vi "Is SPI Channel Ready for Next Transaction.vi"(8 "error in":errorcluster, 11 "Private Data In":T1={"DLU To SPI Engine Data FIFO"="DLU To SPI Engine Data", "SPI Engine to DLU Data FIFO"="SPI Engine to DLU Data", "Data to SPI Engine (Cache) Register"="Data to SPI Engine (Cache)", "SPI PHY Settings to SPI Engine (Cahche) Register"="SPI PHY Settings to SPI Engine (Cache)"}) -> (0 "error out":errorcluster, 1 "SPI Channel Ready":bool, 3 "Private Data Out":T1={"DLU To SPI Engine Data FIFO"="DLU To SPI Engine Data", "SPI Engine to DLU Data FIFO"="SPI Engine to DLU Data", "Data to SPI Engine (Cache) Register"="Data to SPI Engine (Cache)", "SPI PHY Settings to SPI Engine (Cahche) Register"="SPI PHY Settings to SPI Engine (Cache)"}, 4 "Number of Elements to Write":u32)   [LabVIEW 2014]
doc: "This VI reports if SPI Engine is ready to accept new command for SPI Transaction. The SPI Channel Ready output will turn true when the SPI Engine is ready to recieve new data."
uses:
  Controls/Internal Data (SPI API).ctl
  <vilib>/rvi/Emulation/niFpgaSctlEmulationGetInTimedLoop.vi
  <vilib>/rvi/DataTransferAndStorage/Container/Common/niFpgaContainerExecOnDevCompGetState.vi
  <vilib>/rvi/Emulation/niFpgaEmulationIsFPGAContextNoSignature.vi
  <vilib>/rvi/errors/niFpgaSetErrorForExecOnDevCompSimple.vi
  <vilib>/rvi/eio/common/nirviEmuReportErrorAndStop.vi
  <vilib>/rvi/DataTransferAndStorage/Container/Common/niFpgaContainerGetUniqueNameForEmu.vi
  <vilib>/rvi/FIFO/Fifo_Resource/nirvififoEmulationSetSize.vi
  <vilib>/rvi/FIFO/Fifo_Resource/nirviFifoEmulationQueueMgr.vi
  <instcachedir>/0/nirviFifoEmulationQueueMgr_E5CAEC123FF24DC58D834DCA3CDAA9B5.lvgen/nirviFifoEmulationQueueMgr_E5CAEC123FF24DC58D834DCA3CDAA9B5_001.vi
  <vilib>/rvi/FIFO/Fifo_Resource/nirvififoEmulationDetermineInputValidOut.vi
  <vilib>/rvi/FIFO/Fifo_Resource/nirvififoEmulationCreateLock.vi
  <vilib>/rvi/Emulation/niFpgaProcessEmulError.vi
  <vilib>/rvi/FIFO/Fifo_Resource/nirvififoEmulationObtainLock.vi
  <vilib>/rvi/FIFO/Fifo_Resource/nirvififoEmulationReleaseLock.vi
  <vilib>/rvi/occurrence/nirviWaitOnOccurrenceBase.vi
  <vilib>/rvi/errors/nirviReportUnexpectedCaseInternalError.vi
  <vilib>/rvi/errors/nirviReportUnexpectedCaseInternalError (U32).vi
  <vilib>/rvi/interface/RandomDataEmulation/niFpgaRandomDataHandleErrors.vi
  <vilib>/rvi/DataTransferAndStorage/Container/XNode/niFpgaContainer.xnode
  <vilib>/rvi/FIFO/Fifo_Resource/niFpgaFifoEmulationRefIn.vi
panel:
  # "s"
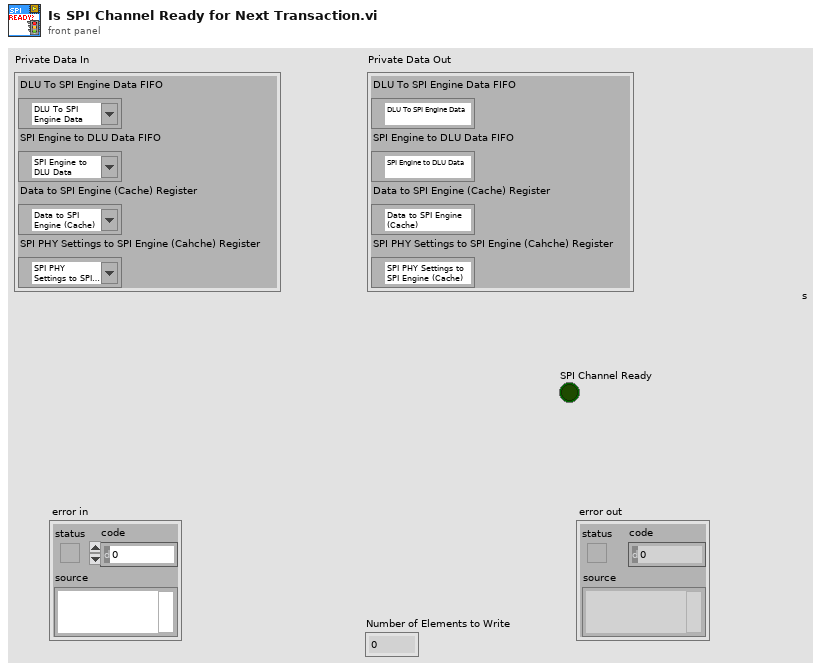
[diagram p1: front panel]
types:
  T1 = typedef "Internal Data (SPI API).ctl" = cluster{"DLU To SPI Engine Data FIFO":refnum<k21>, "SPI Engine to DLU Data FIFO":refnum<k21>, "Data to SPI Engine (Cache) Register":refnum<k21>, "SPI PHY Settings to SPI Engine (Cahche) Register":refnum<k21>}
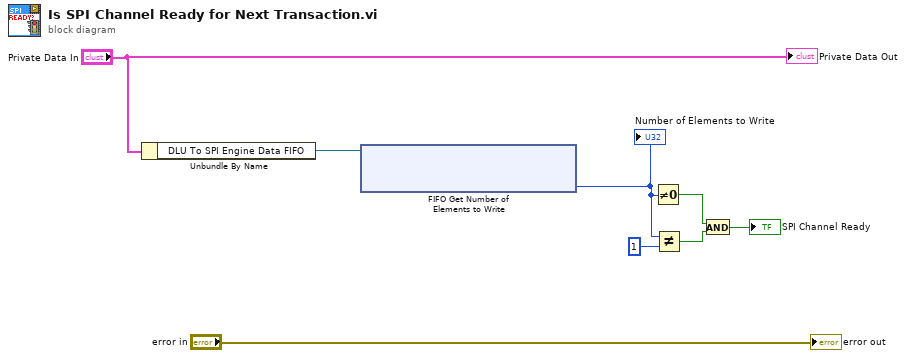
[diagram p0: block diagram]
diagram:
  n1 = Unbundle By Name("Private Data In") -> ("DLU To SPI Engine Data FIFO"=w1:refnum<k21>)
  n2 = xnode "FIFO Get Number of Elements to Write"("FIFO In"=w1) -> ("Number of Elements to Write"=w7:u32)  [unwired: 1 out]
  "Number of Elements to Write" <- w7
  n3 = Not Equal To 0?(x=w7) -> (x != 0?=w5:bool)
  n4 = Not Equal?(x=w7, y=u32 1) -> (x != y?=w6:bool)
  n5 = And(x=w5, y=w6) -> (x .and. y?=→"SPI Channel Ready":bool)
  "Private Data Out" <- "Private Data In"
  "error out" <- "error in"
